vi "RIO and DAC defaults global.vi"() -> ()   [LabVIEW 2017]
panel:
  in  "DAC default enables 3":bool[](array[boolean])=[FALSE, FALSE, FALSE, FALSE, FALSE, FALSE, FALSE, FALSE]
  in  "DAC channel default discription 3":string[](array[string])=["", "", "", "", "", "", "", "\n"]
  in  "DAC default volts 3":dbl[](array[numeric])=[0.0, 0.0, 0.0, 0.0, 0.0, 0.0, 0.0, 0.0]
  in  "Line 3":i32=31
  in  "Port 3":i32=3
  in  "Static DAC device # 3":i16=5
  in  "Port D default discription":string[](array[string])=["", "", "", "", "", "", "", "", "", "", "", "", "", "", "", "", "", "", "", "", "", "", "", "", "", "", "", "", "", "", "", " "]
  in  "Port D default outputs":bool[](array[boolean])=[FALSE, FALSE, FALSE, FALSE, FALSE, FALSE, FALSE, FALSE, FALSE, FALSE, FALSE, FALSE, FALSE, FALSE, FALSE, FALSE, FALSE, FALSE, FALSE, FALSE, FALSE, FALSE, FALSE, FALSE, FALSE, FALSE, FALSE, FALSE, FALSE, FALSE, FALSE, FALSE]
  in  "Port C default discription":string[](array[string])=["", "", "", "", "", "", "", "", "", "", "", "", "", "", "", "", "", "", "", "", "", "", "", "", "", " ", "", "", "", "", "", " "]
  in  "Port C default outputs":bool[](array[boolean])=[FALSE, FALSE, FALSE, FALSE, FALSE, FALSE, FALSE, FALSE, FALSE, FALSE, FALSE, FALSE, FALSE, FALSE, FALSE, FALSE, FALSE, FALSE, FALSE, FALSE, FALSE, FALSE, FALSE, FALSE, FALSE, FALSE, FALSE, FALSE, FALSE, FALSE, FALSE, FALSE]
  in  "Port B default discription":string[](array[string])=["", "", "", "", "", "", "", "", "", "", "", "", "", "", "", "", "", "", "", "", "", "", "", "", "", " ", "", "", "", "", "", "0"]
  in  "Port B default outputs":bool[](array[boolean])=[FALSE, FALSE, FALSE, FALSE, FALSE, FALSE, FALSE, FALSE, FALSE, FALSE, FALSE, FALSE, FALSE, FALSE, FALSE, FALSE, FALSE, TRUE, FALSE, FALSE, FALSE, FALSE, FALSE, FALSE, FALSE, FALSE, FALSE, FALSE, FALSE, FALSE, FALSE, FALSE]
  in  "Port A default discription":string[](array[string])=["", "", "", "", "", "", "", "", "", "", "", "", "", "", "", "", "", "", "", "", "", "", "", "", "", " ", "", "", "", "", "", "0"]
  in  "TTL pulse duration (ms)":dbl=0.001
  in  "Static DAC scale factor":dbl=1.0
  in  "Dynamic DAC device #":i16=6
  in  "Line 2":i32=30
  in  "Port 2":i32=3
  in  "Static DAC device # 2":i16=4
  in  "Line":i32=29
  in  "Port":i32=3
  in  "Static DAC device #":i16=3
  in  "Port A default outputs":bool[](array[boolean])=[FALSE, FALSE, FALSE, FALSE, TRUE, FALSE, FALSE, FALSE, FALSE, TRUE, FALSE, FALSE, FALSE, FALSE, TRUE, FALSE, FALSE, FALSE, FALSE, TRUE, FALSE, FALSE, FALSE, FALSE, TRUE, FALSE, FALSE, FALSE, FALSE, FALSE, FALSE, FALSE]
  in  "DAC default enables 2":bool[](array[boolean])=[FALSE, FALSE, FALSE, FALSE, FALSE, FALSE, FALSE, FALSE]
  in  "DAC default enables 1":bool[](array[boolean])=[FALSE, TRUE, FALSE, FALSE, FALSE, FALSE, FALSE, TRUE]
  in  "DAC channel default discription 2":string[](array[string])=["", "", "", "", "", "", "", "\n"]
  in  "DAC channel default discription 1":string[](array[string])=["aaa", "", "", "", "", "", "", " \n"]
  in  "DAC default volts 2":dbl[](array[numeric])=[0.0, 0.0, 0.0, 0.0, 0.0, 0.0, 0.0, 0.0]
  in  "DAC default volts 1":dbl[](array[numeric])=[0.0, 0.0, 0.0, 3.0, 0.0, 0.0, 0.0, 0.0]
  # "Set up for 2 \"Static\" DAC boards"
  # "0"
  # "TTL trigger for Static DAQ board"
  # "1"
  # "2"
  # "3"
  # "4"
  # "16"
  # "5"
  # "17"
  # "TTL trigger for Static DAQ board"
  # "6"
  # "18"
  # "7"
  # "19"
  # "20"
  # "8"
  # "21"
  # "9"
  # "22"
  # "TTL trigger for Static DAQ board"
  # "10"
  # "23"
  # "11"
  # "12"
  # "13"
  # "14"
  # "15"
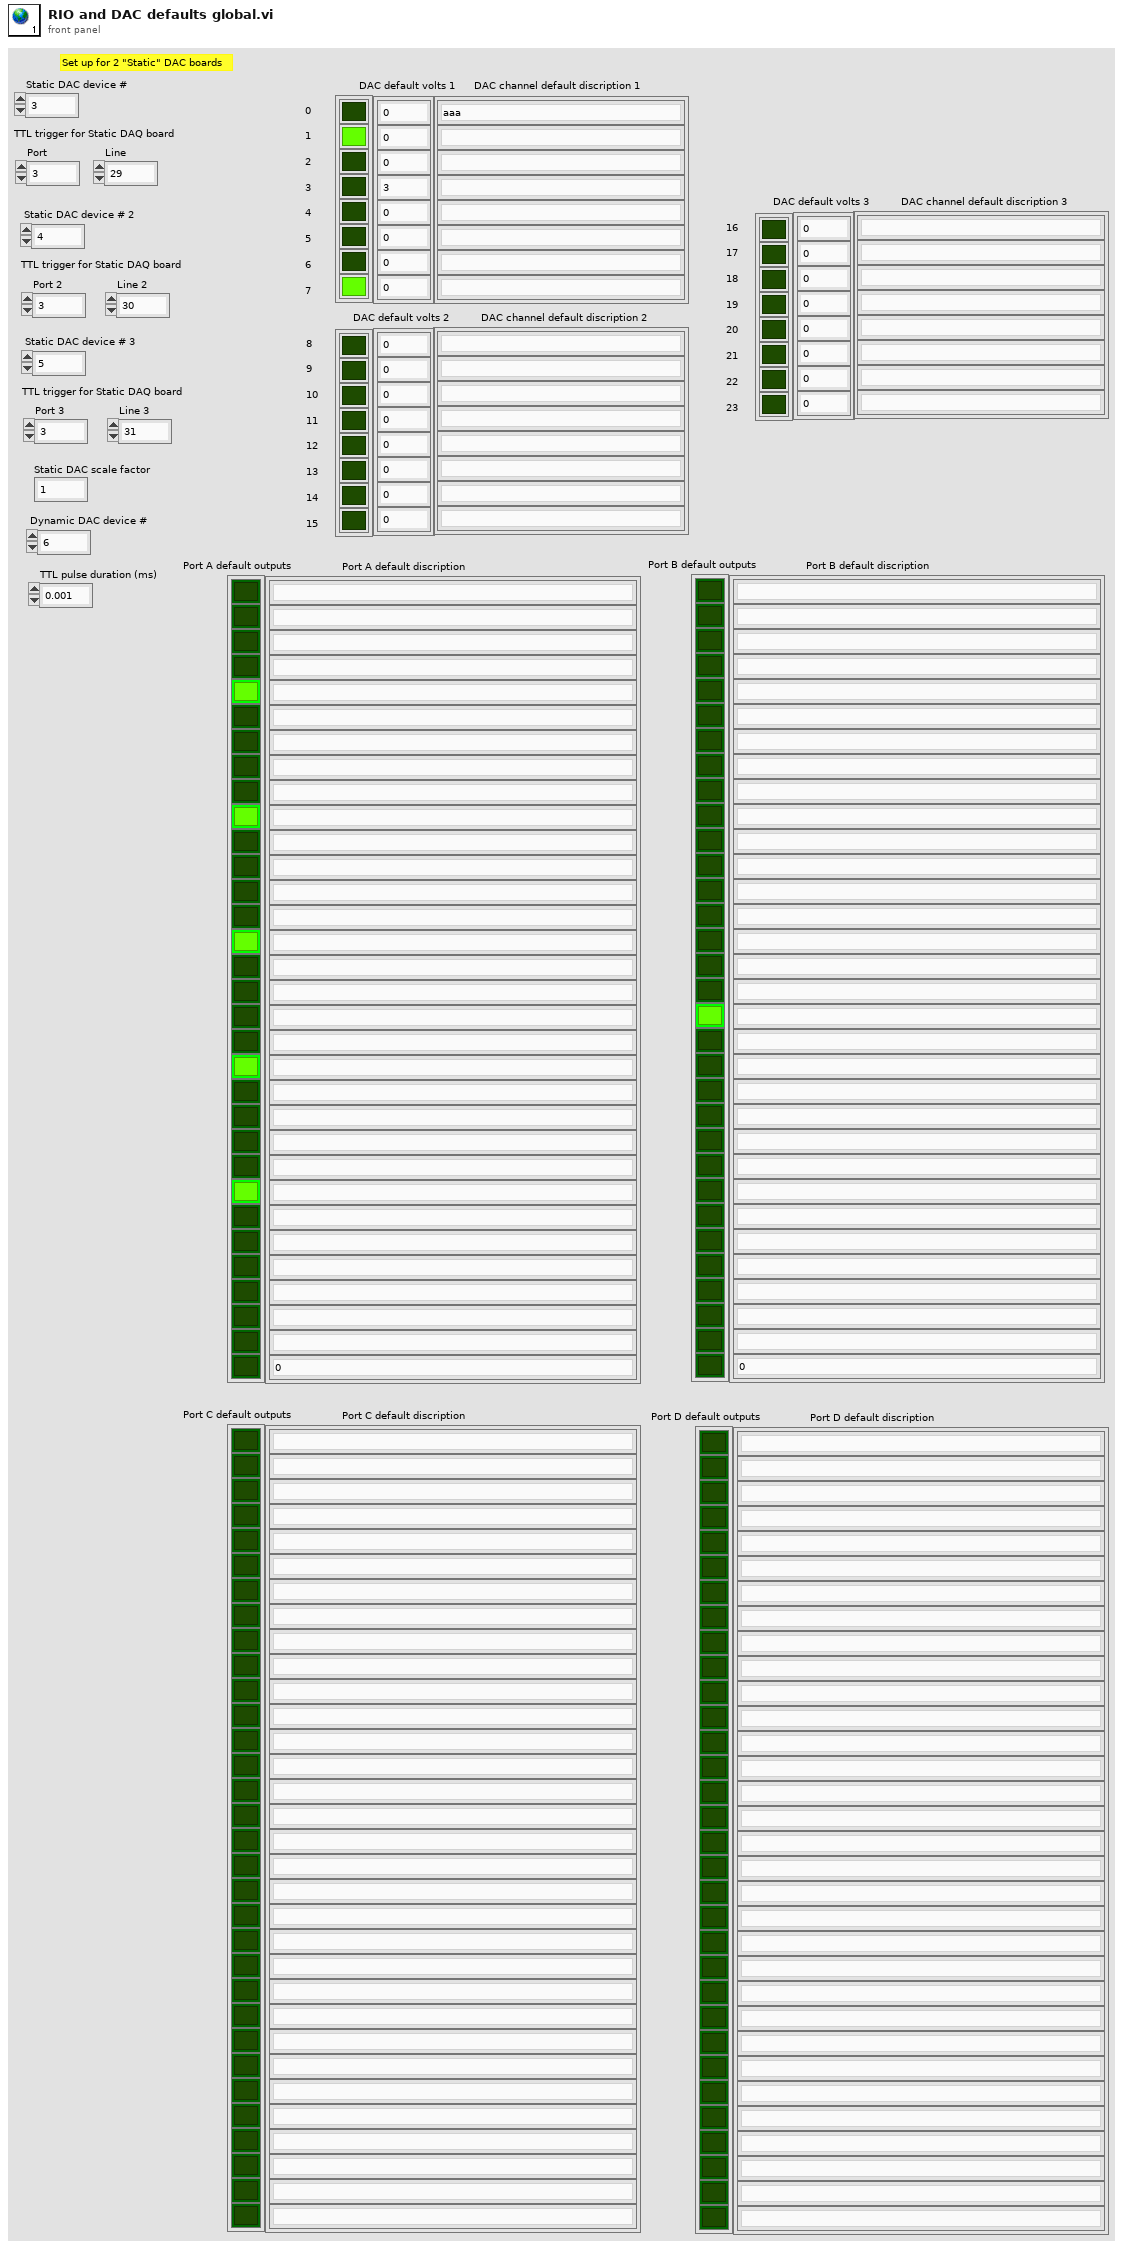
[diagram p1: front panel]
diagram:
